vi "Control Triton Temp 0-2K.vi"(7 "Target Temperature K":dbl, 8 "error in (no error)":errorcluster, 10 "Temp Chan":string="T8", 11 "IP Address":string="128.174.164.8") -> (0 "error out":errorcluster)   [LabVIEW 2018]
panel:
  out "Heater range mA":string
  # "This VI only works and assume the Fridge is running at 0-2K temperature.\nIt will TURN ON/OFF turbo pump of the Triton fridge according to the temperature."
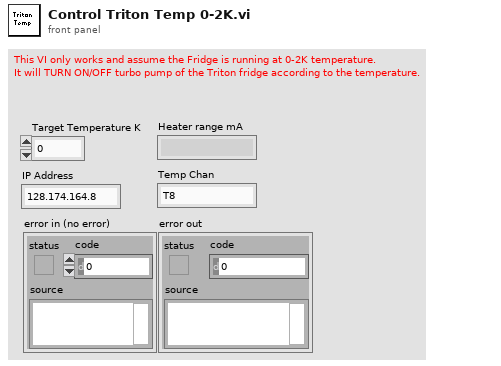
[diagram p1: front panel]
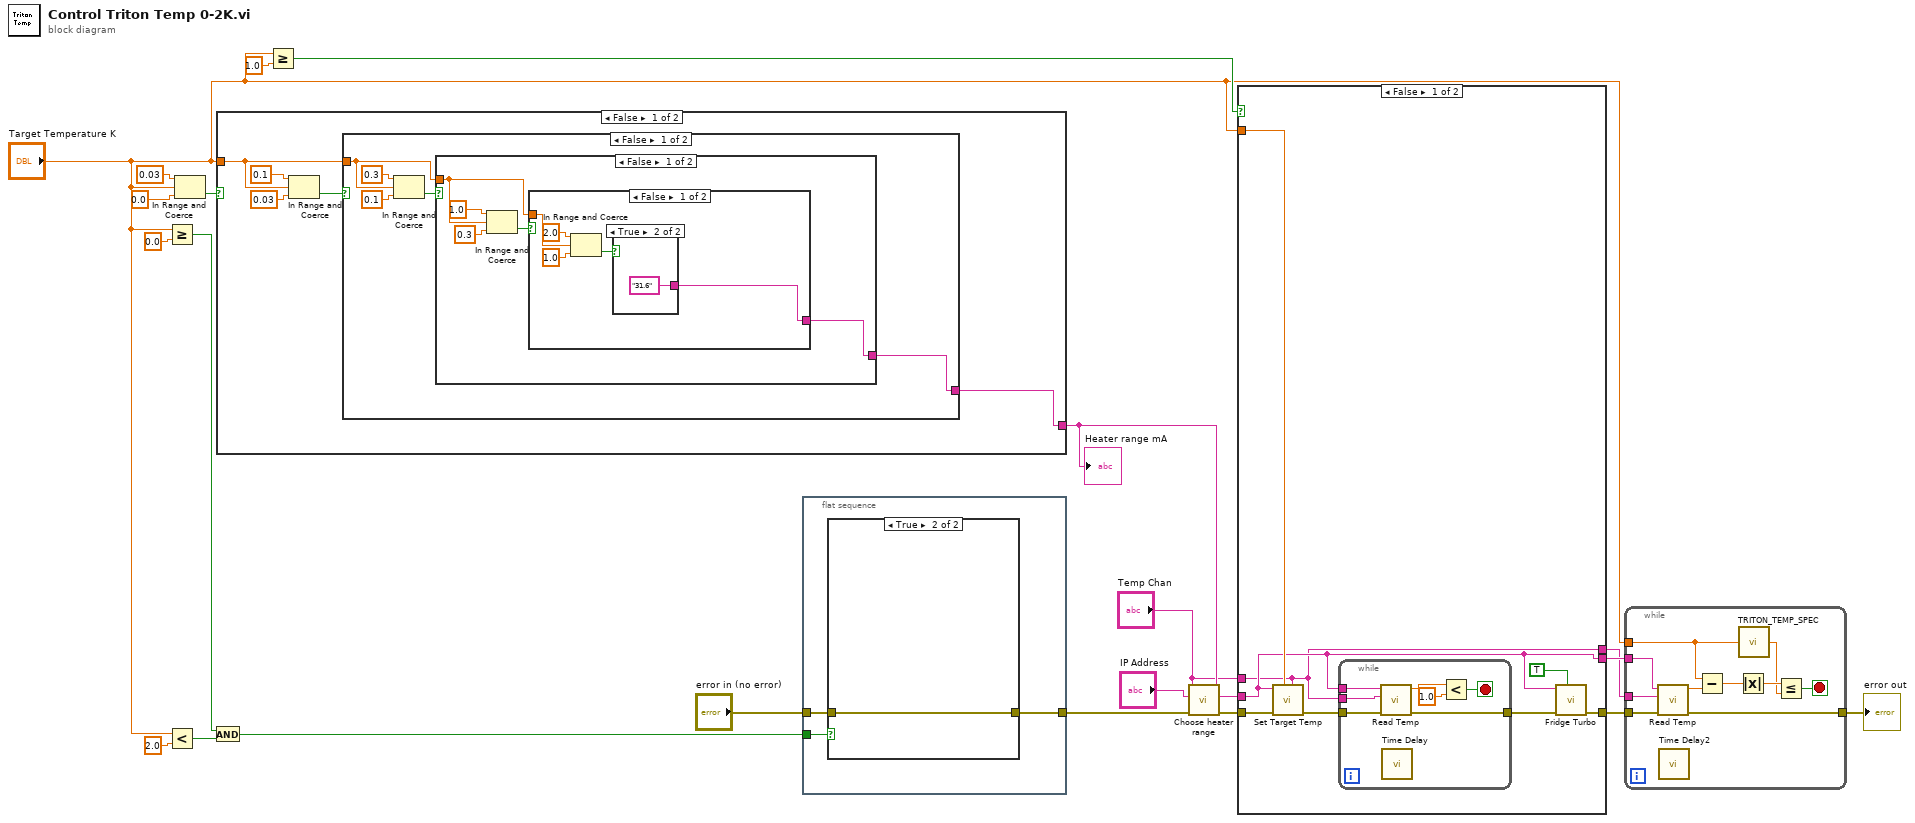
[diagram p0: block diagram]
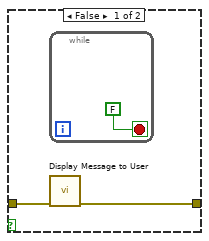
[diagram p2: hidden frame]
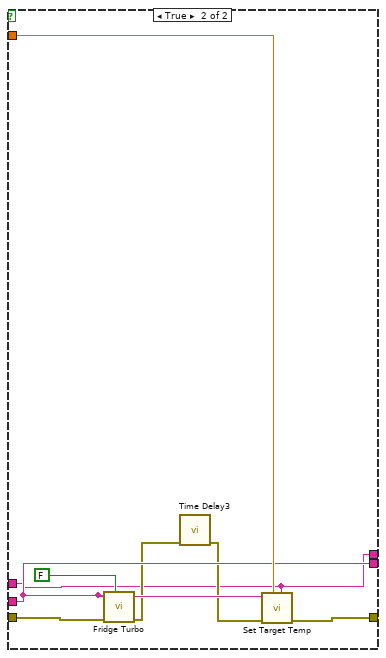
[diagram p3: hidden frame]
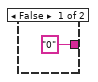
[diagram p4: hidden frame]
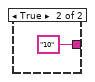
[diagram p5: hidden frame]
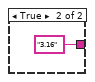
[diagram p6: hidden frame]
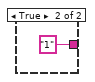
[diagram p7: hidden frame]
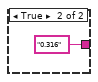
[diagram p8: hidden frame]
diagram:
  n1 = Greater Or Equal?(x="Target Temperature K", y=0.0) -> (x >= y?=w11:bool)
  n2 = Less?(x="Target Temperature K", y=2.0) -> (x < y?=w10:bool)
  n3 = In Range and Coerce(upper limit=0.03, x="Target Temperature K", lower limit=0.0) -> (In Range?=w20:bool)  [unwired: 1 out]
  n4 = And(x=w11, y=w10) -> (x .and. y?=w8:bool)
  n5 = case shown="False" w20 {
    tunnel: [w24 "0.316"] -> w3
    tunnel: "Target Temperature K" -> [w23 _]
    frame False {
      n6 = In Range and Coerce(upper limit=0.1, x=w23, lower limit=0.03) -> (In Range?=w25:bool)  [unwired: 1 out]
      n7 = case shown="False" w25 {
        tunnel: [w29 "1"] -> w24
        tunnel: w23 -> [w28 _]
        frame False {
          n8 = In Range and Coerce(upper limit=0.3, x=w28, lower limit=0.1) -> (In Range?=w30:bool)  [unwired: 1 out]
          n9 = case shown="False" w30 {
            tunnel: [w34 "3.16"] -> w29
            tunnel: w28 -> [w33 _]
            frame False {
              n10 = In Range and Coerce(upper limit=1.0, x=w33, lower limit=0.3) -> (In Range?=w35:bool)  [unwired: 1 out]
              n11 = case shown="False" w35 {
                tunnel: [w38 "10"] -> w34
                tunnel: w33 -> [w40 _]
                frame False {
                  n12 = In Range and Coerce(upper limit=2.0, x=w40, lower limit=1.0) -> (In Range?=w39:bool)  [unwired: 1 out]
                  n13 = case shown="True" w39 {
                    tunnel: ["0" "31.6" ("lower limit")] -> w38
                    frame False {
                    }
                    frame True {
                    }
                  }
                }
                frame True {
                }
              }
            }
            frame True {
            }
          }
        }
        frame True {
        }
      }
    }
    frame True {
    }
  }
  "Heater range mA" <- w3
  n14 = Greater Or Equal?(x="Target Temperature K", y=1.0) -> (x >= y?=w18:bool)
  n15 = flat-sequence {
    tunnel: "error in (no error)" -> [w50]
    tunnel: [w49] -> w13
    tunnel: w8 -> [w51]
    frame #0 {
      n16 = case shown="True" w51 {
        tunnel: w50 -> [w53 w55]
        tunnel: [w52 w55] -> w49
        frame False {
          n17 = while {
            stop <- FALSE stop-if-true
          }
          n18 = call "Display Message to User"("error in (no error)"=w53) -> ("error out"=w52:errorcluster)  [unwired: 9 in, 1 out]
        }
        frame True {
        }
      }
    }
  }
  n19 = call "Choose heater range.vi"("Heater range mA"=w3, "error in (no error)"=w13, "IP Address in"="IP Address", "Temp Chan"="Temp Chan") -> ("error out"=w17:errorcluster, "IP Address out"=w16:string)  [unwired: 6 in]
  n20 = case shown="False" w18 {
    tunnel: w17 -> [w61 w78]
    tunnel: w16 -> [w57 w74]
    tunnel: "Target Temperature K" -> [w59 w76]
    tunnel: [w58 w75] -> w7
    tunnel: [w57 w74] -> w6
    tunnel: "Temp Chan" -> [w56 w71]
    tunnel: [w56 w71] -> w1
    frame False {
      n21 = call "Set Target Temp.vi"("Temp Chan"=w56, "T Set"=w59, "error in (no error)"=w61, "IP Address in"=w57) -> ("error out"=w60:errorcluster)  [unwired: 7 in]
      n22 = while {
        tunnel: w57 -> [w70]
        tunnel: w60 -> [w69]
        tunnel: [w65] -> w63
        tunnel: w56 -> [w64]
        stop <- w66 stop-if-true
        n23 = call "Read Temp.vi"("error in (no error)"=w69, "Temp Chan"=w64, "IP Address in"=w70) -> ("error out"=w65:errorcluster, "Temperature"=w68:dbl)  [unwired: 7 in]
        n24 = call "Time Delay"() -> ()  [unwired: 11 in, 1 out]
        n25 = Less?(x=w68, y=1.0) -> (x < y?=w66:bool)
      }
      n26 = call "Fridge Turbo.vi"("On OFF"=TRUE, "error in (no error)"=w63, "IP Address in"=w57) -> ("error out"=w58:errorcluster)  [unwired: 8 in]
    }
    frame True {
      n27 = call "Fridge Turbo.vi"("On OFF"=FALSE, "error in (no error)"=w78, "IP Address in"=w74) -> ("error out"=w73:errorcluster)  [unwired: 8 in]
      n28 = call "Time Delay3"("error in (no error)"=w73) -> ("error out"=w72:errorcluster)  [unwired: 10 in]
      n29 = call "Set Target Temp.vi"("Temp Chan"=w71, "T Set"=w76, "error in (no error)"=w72, "IP Address in"=w74) -> ("error out"=w75:errorcluster)  [unwired: 7 in]
    }
  }
  n30 = while {
    tunnel: w7 -> [w88]
    tunnel: w6 -> [w87]
    tunnel: "Target Temperature K" -> [w83]
    tunnel: [w80] -> w4
    tunnel: w1 -> [w79]
    stop <- w81 stop-if-true
    n31 = call "Read Temp.vi"("error in (no error)"=w88, "Temp Chan"=w79, "IP Address in"=w87) -> ("error out"=w80:errorcluster, "Temperature"=w86:dbl)  [unwired: 7 in]
    n32 = call "Time Delay2"() -> ()  [unwired: 11 in, 1 out]
    n33 = Subtract(x=w83, y=w86) -> (x-y=w85:dbl)
    n34 = Absolute Value(x=w85) -> (abs(x)=w84:dbl)
    n35 = call "TRITON_TEMP_SPEC.vi"("Target Temperature [K]"=w83) -> ("Temperature Stability Specification"=w82:dbl)
    n36 = Less Or Equal?(x=w84, y=w82) -> (x <= y?=w81:bool)
  }
  "error out" <- w4
